vi "Close Session.vi"(6 "Target Config":T1={"IP Address"="0.0.0.0", "Target"=enum."cRIO-9012", "Username"="", "Password"=""}, 8 "error in (no error)":errorcluster, 10 "Sys Cfg Session In":refnum<k21>, 11 "Console Ref In":refnum<vi>) -> (0 "error out":errorcluster, 3 "Console Ref Out":refnum<vi>)   [LabVIEW 2015]
doc: "Close system configuration session to the target."
uses:
  Type Defs/Target Config Cluster.ctl
  Type Defs/RT Target Type.ctl
  <vilib>/nisyscfg/Close (System).vi
  <vilib>/nisyscfg/nisyscfg.lvlib
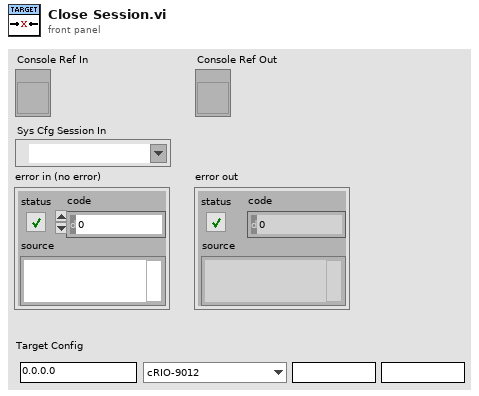
[diagram p1: front panel]
types:
  T1 = typedef "Target Config Cluster.ctl" = cluster{"IP Address":string, "Target":T2, "Username":string, "Password":string}
  T2 = typedef "RT Target Type.ctl" = enum16{"cRIO-9012", "cRIO-9014", "cRIO-9022", "cRIO-9023", "cRIO-9024", "cRIO-9025", "cRIO-9068", "cRIO-9073", "cRIO-9074", "cRIO-9075", "cRIO-9076", "cRIO-9081", "cRIO-9082", "myRIO-1900", "myRIO-1950", "PXI-8101", "PXI-8115", "PXI-8119", "PXI-8820", "PXIe-8100", "PXIe-8101", "PXIe-8133", "PXIe-8135", "PXIe-8820", "sbRIO-9605", "sbRIO-9606", "sbRIO-9623", "sbRIO-9626", "sbRIO-9633", "sbRIO-9636", "Unlisted (Linux-RT)", "Unlisted (PharLap)", "Unlisted (VxWorks)"}
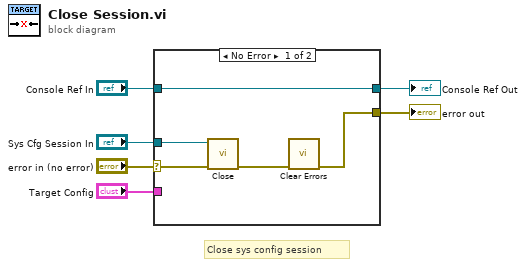
[diagram p0: block diagram]
diagram:
  # "Close sys config session"
  n1 = case shown="No Error" "error in (no error)" {
    selector: "error in (no error)" -> [w10 w12]
    tunnel: "Console Ref In" -> [w8 w13]
    tunnel: "Target Config" -> [_ _]
    tunnel: [w8 w13] -> w3
    tunnel: [w7 w12] -> w2
    tunnel: "Sys Cfg Session In" -> [w11 _]
    frame No Error {
      n2 = call-poly <vilib>:"Close.vi"("error in (no error)"=w10, "Session in"=w11) -> ("error out"=w9:errorcluster)  [unwired: 9 in]
      n3 = call <vilib>:"Clear Errors.vi"("error in (no error)"=w9) -> ("error out"=w7:errorcluster)  [unwired: 5 in, 1 out]
    }
    frame Error {
    }
  }
  "error out" <- w2
  "Console Ref Out" <- w3
